vi "Create Close Reference VIs.vi"   [LabVIEW 2015]
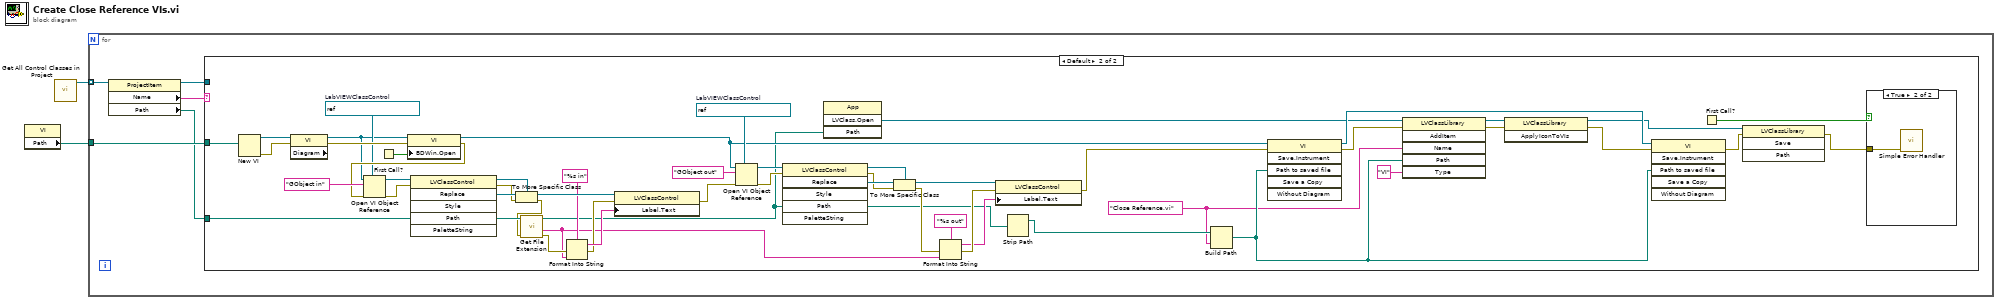
[diagram p0: block diagram]
diagram:
  n1 = property class="VI"() -> ("Path"=w1:path)  [unwired: 2 in, 2 out]
  n2 = call "Get All Control Classes in Project.vi"() -> ("All Control Classes"=w2:refnum<vi>[])  [unwired: 11 in]
  n3 = for {
    tunnel: w2 -> [w7] mode=indexing
    tunnel: w1 -> [w4]
    n4 = property class="ProjectItem"(reference=w7) -> (reference out=w5:refnum<vi>, "Name"=w6:string, "Path"=w3:path)  [unwired: 1 in, 1 out]
    n5 = case shown="Default" w6 {
      tunnel: w5 -> [_ _]
      tunnel: w4 -> [_ w59]
      tunnel: w3 -> [_ w44]
      frame "GObject.lvclass", "Generic.lvclass" {
      }
      frame Default {
        w10 = "Close Reference.vi"
        w19 = refnum<vi> refnum  # LabVIEWClassControl
        w55 = refnum<vi> refnum  # LabVIEWClassControl
        n6 = New VI(10:w59) -> (0:w50:errorcluster, 3:w58:refnum<vi>)  [unwired: 6 in]
        n7 = property class="VI" props=["Diagram"](reference=w58, error in=w50) -> (reference out=w15:refnum<vi>, error out=w49:errorcluster)  [unwired: 1 out]
        n8 = First Call?() -> (First Call?: T/F=w21:bool)
        n9 = property class="VI"(reference=w15, error in=w49, "BDWin.Open"=w21) -> (reference out=w28:refnum<vi>, error out=w48:errorcluster)
        n10 = Open VI Object Reference(7:w19, 8:w48, 10:"GObject in" ("name/order"), 11:w15) -> (0:w51:errorcluster, 3:w56:refnum<vi>)
        n11 = invoke class="LVClassControl" method="Replace"(reference=w56, error in=w51, "Path"=w44) -> (reference out=w45:refnum<vi>, error out=w39:errorcluster, "Replace"=w47:refnum<vi>)  [unwired: 3 in, 3 out]
        n12 = To More Specific Class(target class=w45, reference=w47, error in=w39) -> (specific class reference=w46:refnum<vi>, error out=w38:errorcluster)
        n13 = call <vilib>:"Get File Extension.vi"("error in (no error)"=w38, "file"=w44) -> ("error out"=w37:errorcluster, "filename without extension"=w8:string, "dup file"=w27:path)  [unwired: 5 in, 2 out]
        n14 = Format Into String(format string="%s in", error in=w37, w8) -> (resulting string=w42:string, error out=w36:errorcluster)  [unwired: 1 in]
        n15 = property class="LVClassControl"(reference=w46, error in=w36, "Label.Text"=w42) -> (error out=w35:errorcluster)  [unwired: 1 out]
        n16 = Open VI Object Reference(7:w55, 8:w35, 10:"GObject out" ("name/order"), 11:w28) -> (0:w52:errorcluster, 3:w53:refnum<vi>)
        n17 = invoke class="LVClassControl" method="Replace"(reference=w53, error in=w52, "Path"=w27) -> (reference out=w40:refnum<vi>, error out=w34:errorcluster, "Replace"=w41:refnum<vi>)  [unwired: 3 in, 3 out]
        n18 = invoke class="App" method="LVClass.Open"("Path"=w27) -> ("LVClass.Open"=w9:refnum<vi>)  [unwired: 3 in, 3 out]
        n19 = To More Specific Class(target class=w40, reference=w41, error in=w34) -> (specific class reference=w31:refnum<vi>, error out=w33:errorcluster)
        n20 = Format Into String(format string="%s out", error in=w33, w8) -> (resulting string=w29:string, error out=w30:errorcluster)  [unwired: 1 in]
        n21 = property class="LVClassControl"(reference=w31, error in=w30, "Label.Text"=w29) -> (error out=w18:errorcluster)  [unwired: 1 out]
        n22 = Strip Path(path=w27) -> (stripped path=w26:path)  [unwired: 1 out]
        n23 = Build Path(base path=w26, name or relative path=w10) -> (appended path=w14:path)
        n24 = invoke class="VI" method="Save.Instrument"(reference=w28, error in=w18, "Path to saved file"=w14) -> (reference out=w16:refnum<vi>, error out=w25:errorcluster)  [unwired: 3 in, 4 out]
        n25 = invoke class="LVClassLibrary" method="AddItem"(reference=w9, error in=w25, "Name"=w10, "Path"=w14, "Type"="VI") -> (reference out=w23:refnum<vi>, error out=w22:errorcluster)  [unwired: 1 in, 4 out]
        n26 = invoke class="LVClassLibrary" method="ApplyIconToVIs"(reference=w23, error in=w22) -> (reference out=w13:refnum<vi>, error out=w17:errorcluster)  [unwired: 1 in, 1 out]
        n27 = invoke class="VI" method="Save.Instrument"(reference=w16, error in=w17, "Path to saved file"=w14) -> (error out=w12:errorcluster)  [unwired: 3 in, 5 out]
        n28 = First Call?() -> (First Call?: T/F=w20:bool)
        n29 = invoke class="LVClassLibrary" method="Save"(reference=w13, error in=w12) -> (error out=w11:errorcluster)  [unwired: 2 in, 3 out]
        n30 = case shown="True" w20 {
          tunnel: w11 -> [_ w60]
          frame False {
          }
          frame True {
            n31 = call <vilib>:"Simple Error Handler.vi"("error in (no error)"=w60) -> ()  [unwired: 4 in, 5 out]
          }
        }
      }
    }
  }
